vi "Teleop.vi"(10 "Match Info":T2={"Autonomous Elapsed Seconds"=0.0, "TeleOp Elapsed Seconds"=23.221, "Disabled Elapsed Seconds"=215.834, "Visited Autonomous"=FALSE, "Visited TeleOp"=TRUE, "Visited Disabled"=TRUE, "Autonomous Settings"={"Autonomous Style"=enum."Independent", "VI Refnum"=refnum}}, 11 "Call Context":T3=enum."Stop") -> ()   [LabVIEW 2016]
doc: "This VI is called for each TeleOp packet received from the DS where the robot is not disabled. It is often used to read from the joysticks and update I/O or to update setpoints for timed control loops. It should complete and return within 20 milliseconds or it may miss DS packets."
uses:
  <vilib>/Rock Robotics/WPI/DriverStation/WPI_DriverStationDerivedRobotMode.ctl
  <vilib>/Rock Robotics/WPI/DriverStation/WPI_DriverStationMatch Info.ctl
  <userlib>/836-libraries/Drive/Drive_Code/Drive_Code_Support/Drive_Code_PID_Bundle.ctl
  FMS Commands.ctl
  Drive Commands.ctl
  Gear Command.ctl
  <userlib>/836-libraries/Drive/Drive_Code/Drive_Code_Support/Sensor_Cluster.ctl
  <userlib>/836-libraries/Drive/Drive_Code/Drive_Code_Support/Camera_Cluster.ctl
  <userlib>/836-libraries/Drive/Drive_Code/Drive_Code_Support/Drive_Code_Notifier.ctl
  <userlib>/836-libraries/Drive/Drive_Code/Drive_Code_Support/Drive_Code_Command.ctl
  <userlib>/836-libraries/Drive/Drive_Code/Logging_Data.ctl
  <vilib>/Rock Robotics/WPI/Utilities/WPI_GetSetVariantRefNum.vi
panel:
  in  "Tab Control":enum32{"Drive", "Page 2"}(tab)
  in  "High Gear PID":T1={"Yaw, Driving Straight"={"proportional gain (Kc)"=1.0, "integral time (Ti, min)"=0.01, "derivative time (Td, min)"=0.0}, "Yaw, Holding Still"={"proportional gain (Kc)"=1.0, "integral time (Ti, min)"=0.01, "derivative time (Td, min)"=0.0}, "Distance, Driving Straight"={"proportional gain (Kc)"=1.0, "integral time (Ti, min)"=0.01, "derivative time (Td, min)"=0.0}, "Distance, Holding Still"={"proportional gain (Kc)"=1.0, "integral time (Ti, min)"=0.01, "derivative time (Td, min)"=0.0}}
  in  "Low Gear PID":T1={"Yaw, Driving Straight"={"proportional gain (Kc)"=1.0, "integral time (Ti, min)"=0.01, "derivative time (Td, min)"=0.0}, "Yaw, Holding Still"={"proportional gain (Kc)"=1.0, "integral time (Ti, min)"=0.01, "derivative time (Td, min)"=0.0}, "Distance, Driving Straight"={"proportional gain (Kc)"=1.0, "integral time (Ti, min)"=0.01, "derivative time (Td, min)"=0.0}, "Distance, Holding Still"={"proportional gain (Kc)"=1.0, "integral time (Ti, min)"=0.01, "derivative time (Td, min)"=0.0}}
  in  "PID Update":bool
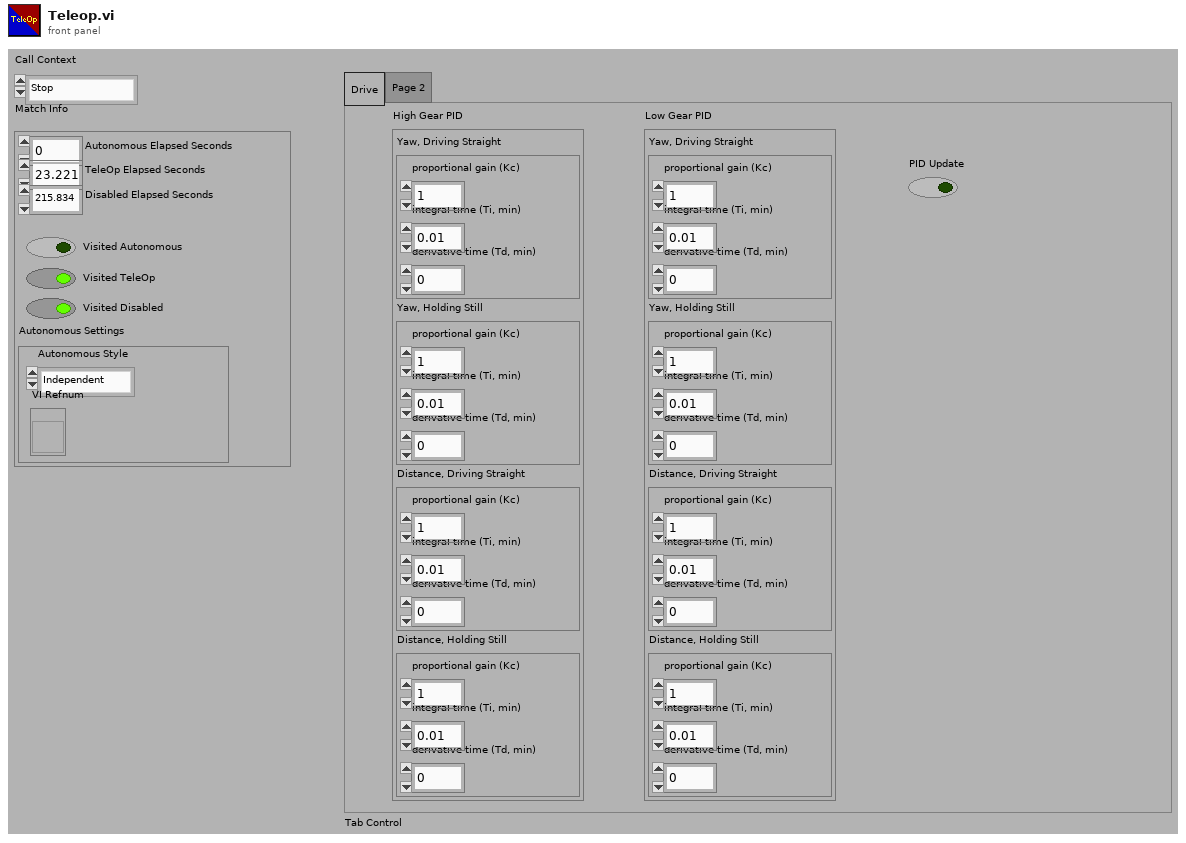
[diagram p1: front panel]
types:
  T1 = typedef "Drive_Code_PID_Bundle.ctl" = cluster{"Yaw, Driving Straight":cluster{"proportional gain (Kc)":dbl, "integral time (Ti, min)":dbl, "derivative time (Td, min)":dbl}, "Yaw, Holding Still":cluster{"proportional gain (Kc)":dbl, "integral time (Ti, min)":dbl, "derivative time (Td, min)":dbl}, "Distance, Driving Straight":cluster{"proportional gain (Kc)":dbl, "integral time (Ti, min)":dbl, "derivative time (Td, min)":dbl}, "Distance, Holding Still":cluster{"proportional gain (Kc)":dbl, "integral time (Ti, min)":dbl, "derivative time (Td, min)":dbl}}
  T2 = typedef "WPI_DriverStationMatch Info.ctl" = cluster{"Autonomous Elapsed Seconds":dbl, "TeleOp Elapsed Seconds":dbl, "Disabled Elapsed Seconds":dbl, "Visited Autonomous":bool, "Visited TeleOp":bool, "Visited Disabled":bool, "Autonomous Settings":cluster{"Autonomous Style":enum16{"Iterative", "Independent"}, "VI Refnum":refnum<vi>}}
  T3 = typedef "WPI_DriverStationDerivedRobotMode.ctl" = enum16{"Init", "Execute", "Stop"}
  T4 = typedef "WPI_JoystickDevRef.ctl" = cluster{"Device":T5}
  T5 = typedef "WPI_JoystickDeviceEnum.ctl" = enum16{"USB 0", "USB 1", "USB 2", "USB 3", "USB 4", "USB 5"}
  T6 = enum8{"setop", "setcolor", "default", "pilot", "ball", "gear", "both", "gearDeliver", "timeWarn", "targeting", "rave", "debug", "Set Power"}
  T7 = typedef "Sensor_Cluster.ctl" = cluster{"Gyro Data":cluster{"Gyro RT FIFO":refnum<k33>, "Gyro Current":dbl, "Gyro Hold":dbl}, "Encoder Data":cluster{"Encoder RT FIFO":refnum<k33>, "Encoder Current":dbl, "Encoder Hold":dbl}, "Camera Data":cluster{"Camera RT FIFO":refnum<k33>, "Camera Current":T8}}
  T8 = typedef "Camera_Cluster.ctl" = cluster{" Angle":dbl, "Valid":bool}
  T9 = cluster{"Cluster":T7, "Drive Command rt fifo":refnum<k33>, "Logging Data":refnum<k33>, "PID Update":refnum<notifier>}
  T10 = typedef "FMS Commands.ctl" = enum16{"Shoot", "Un-Jam", "Stop"}
  T11 = typedef "Gear Command.ctl" = enum16{"Home", "Floor Intake", "Catch", "Score"}
  T12 = typedef "Drive Commands.ctl" = enum16{"Manual", "Get Gear", "Score Gear", "Align Rope", "Turn To Angle", "Start Gear Score", "Place Gear", "Tank Drive", "Drive Distance"}
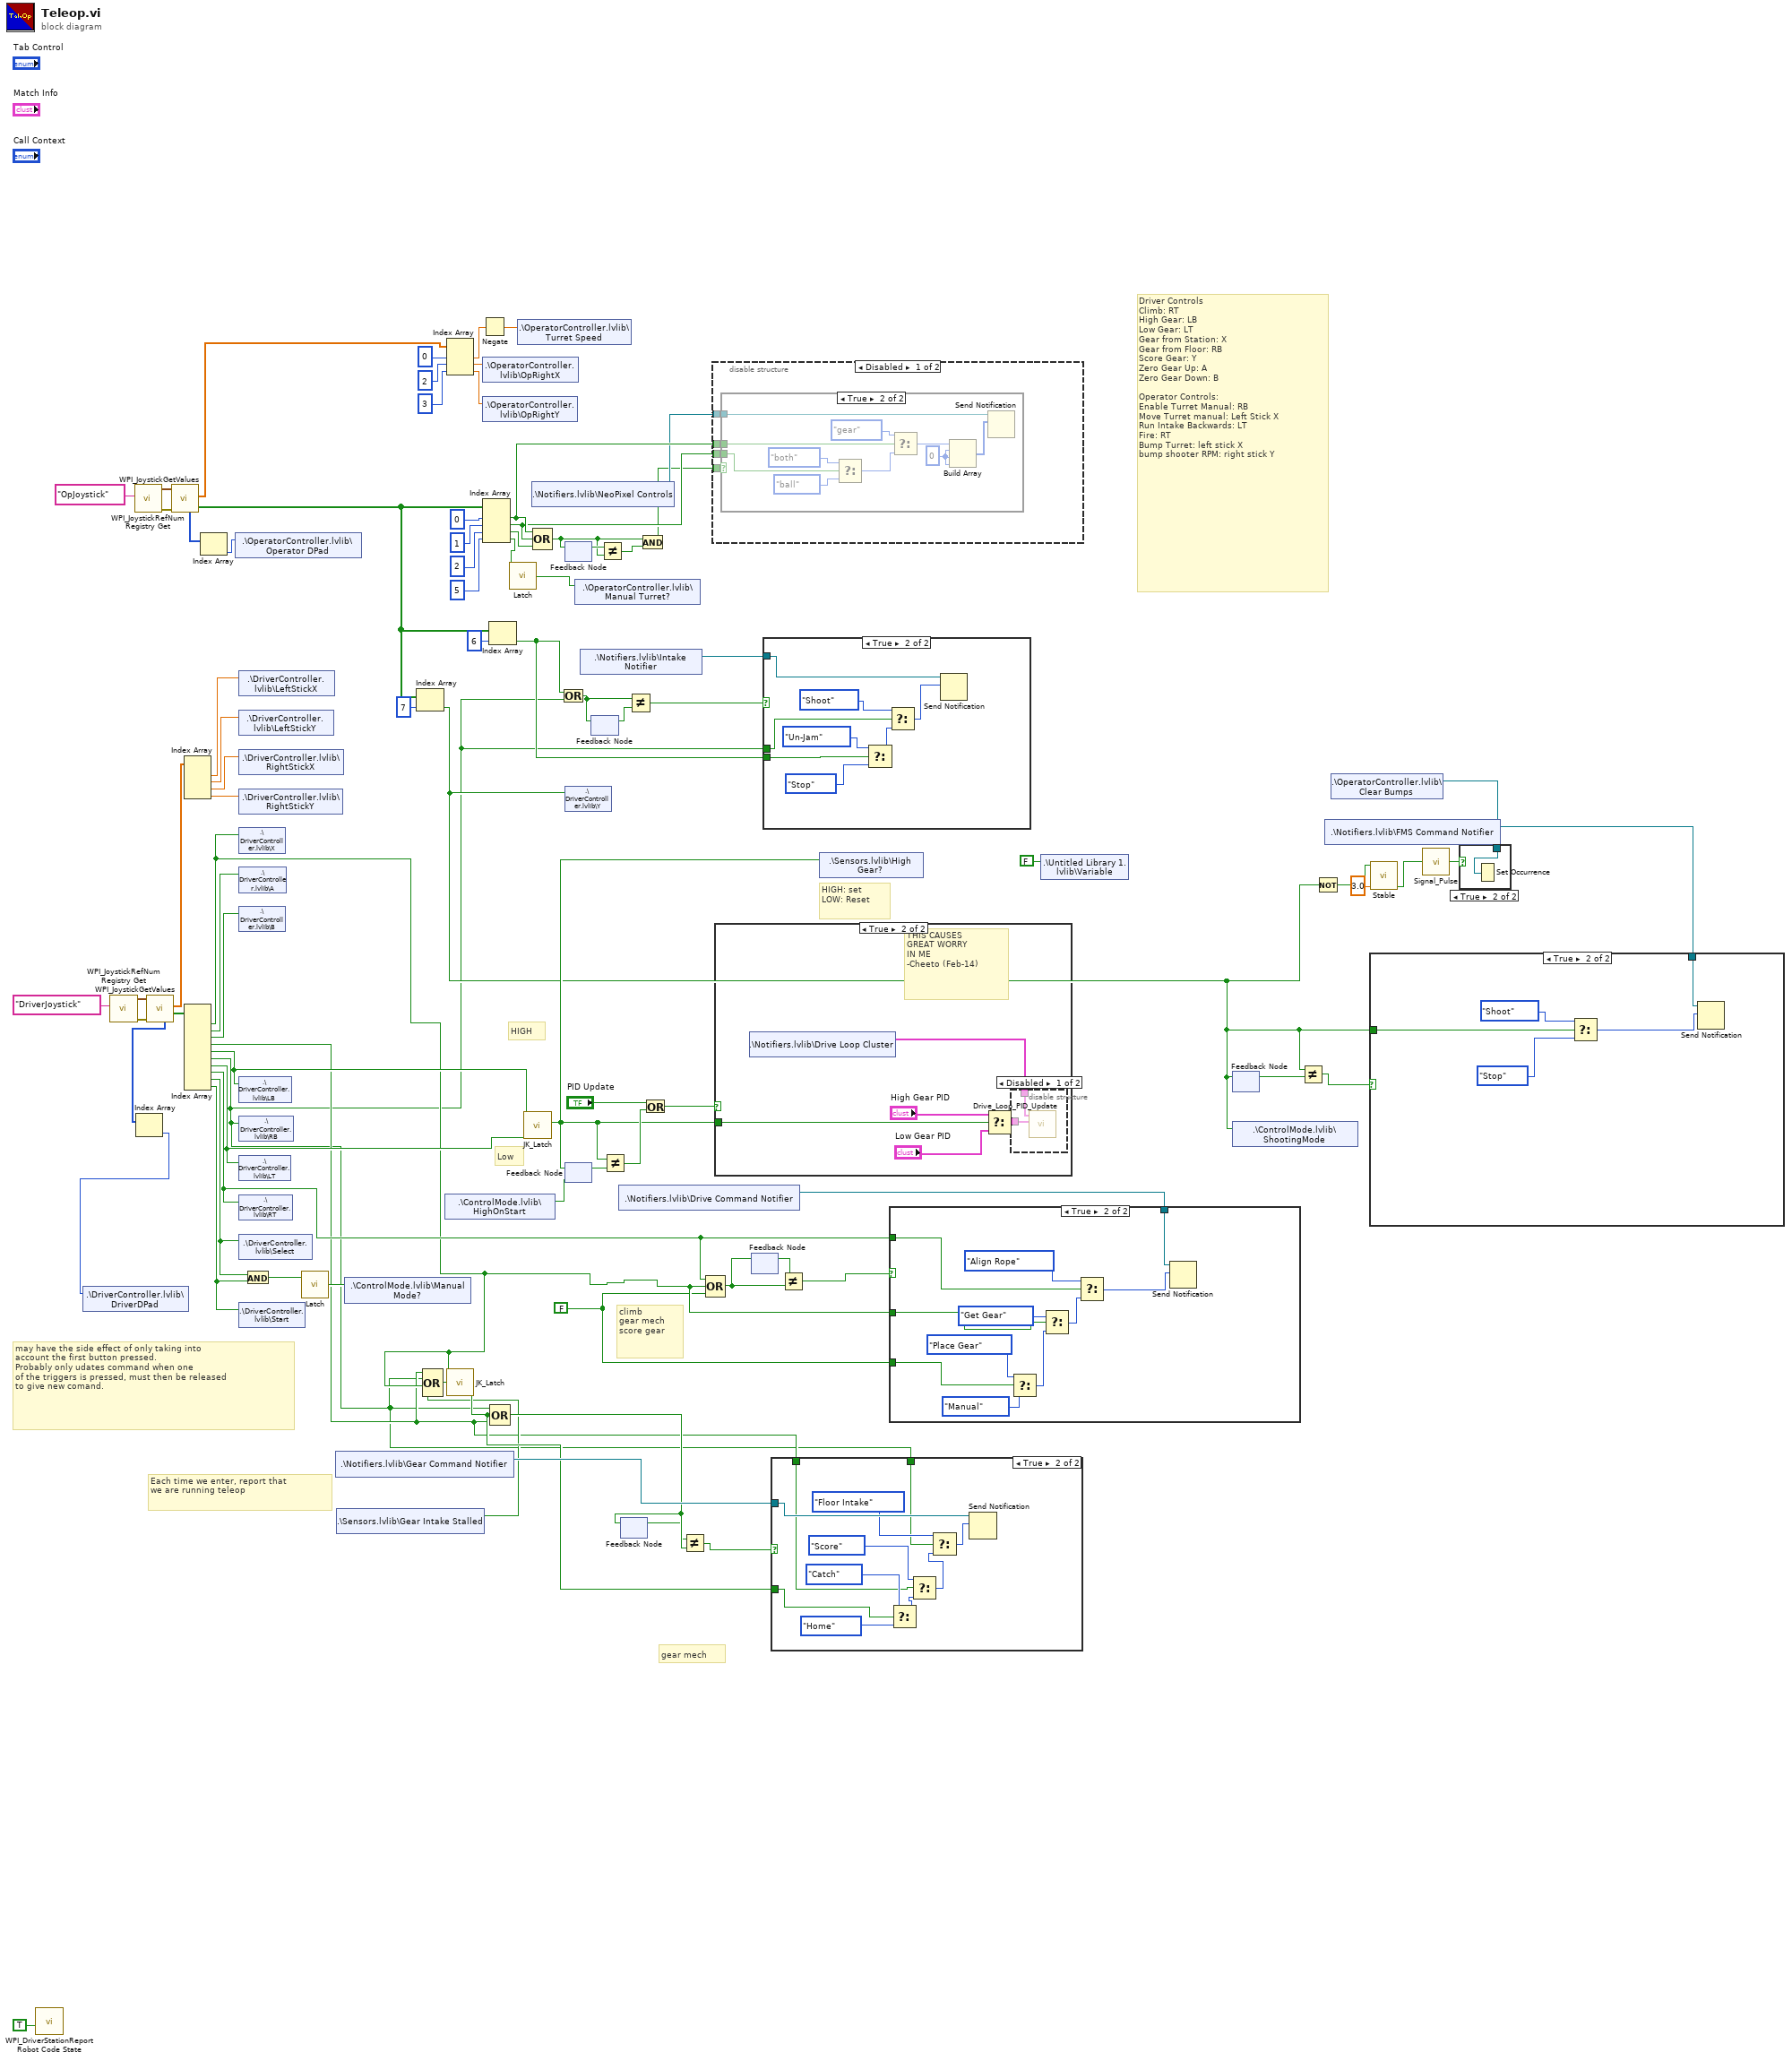
[diagram p0: block diagram]
diagram:
  w1 = FALSE ("value")
  # "climb\ngear mech\nscore gear"
  # "gear mech"
  # "HIGH: set\nLOW: Reset"
  # "Low"
  # "HIGH"
  # "Driver Controls\nClimb: RT\nHigh Gear: LB\nLow Gear: LT\nGear from Station: X\nGear from Floor: RB\nScore Gear: Y\nZero Gear Up: A\nZero Gear Down: B\n\nOperator Controls:\nEnable Turret Manual: RB\nMove Turret manual: Left Stick X\nRun Intake Backwards: LT\nFire: RT\nBump Turret: left stick X\nbump shooter RPM: right stick Y"
  # "may have the side effect of only taking into\naccount the first button pressed.\nProbably only udates command when one\nof the triggers is pressed, must then be released\nto give new comand."
  # "Each time we enter, report that\nwe are running teleop"
  n1 = call <vilib>:"WPI_DriverStationReport Robot Code State.vi"("TeleOp"=TRUE ("Autonomous")) -> ()  [unwired: 10 in, 1 out]
  n2 = call <vilib>:"WPI_JoystickRefNum Registry Get.vi"("refnum name"="DriverJoystick") -> ("error out"=w54:errorcluster, "JoystickDevRef"=w55:T4)  [unwired: 9 in]
  n3 = call <vilib>:"WPI_JoystickRefNum Registry Get.vi"("refnum name"="OpJoystick") -> ("error out"=w68:errorcluster, "JoystickDevRef"=w66:T4)  [unwired: 9 in]
  n4 = call <vilib>:"WPI_JoystickGetValues.vi"("error in (no error)"=w54, "JoystickDevRef"=w55) -> ("Buttons"=w84:bool[], "Axes"=w85:dbl[], "POVs"=w37:i16[])  [unwired: 5 in, 2 out]
  n5 = Index Array(array=w37) -> (element=w36:i16)  [unwired: 1 in]
  n6 = shared-variable ".\\DriverController.lvlib\\DriverDPad"(w36) -> ()  [unwired: 1 in, 1 out]
  n7 = call <vilib>:"WPI_JoystickGetValues.vi"("error in (no error)"=w68, "JoystickDevRef"=w66) -> ("Buttons"=w33:bool[], "Axes"=w65:dbl[], "POVs"=w35:i16[])  [unwired: 5 in, 2 out]
  n8 = Index Array(array=w85) -> (element #1=w83:dbl, element #2=w74:dbl, element #3=w73:dbl, element #4=w82:dbl)  [unwired: 4 in]
  n9 = Index Array(array=w84) -> (element #1=w4:bool, element #2=w14:bool, element #3=w69:bool, element #4=w3:bool, element #5=w48:bool, element #6=w2:bool, element #7=w47:bool, element #8=w15:bool, element #9=w78:bool, element #10=w77:bool)  [unwired: 10 in]
  n10 = Index Array(array=w35) -> (element=w34:i16)  [unwired: 1 in]
  n11 = shared-variable ".\\OperatorController.lvlib\\Operator DPad"(w34) -> ()  [unwired: 1 in, 1 out]
  n12 = shared-variable ".\\DriverController.lvlib\\LeftStickX"(w83) -> ()  [unwired: 1 in, 1 out]
  n13 = shared-variable ".\\DriverController.lvlib\\LeftStickY"(w74) -> ()  [unwired: 1 in, 1 out]
  n14 = shared-variable ".\\DriverController.lvlib\\RightStickX"(w73) -> ()  [unwired: 1 in, 1 out]
  n15 = shared-variable ".\\DriverController.lvlib\\RightStickY"(w82) -> ()  [unwired: 1 in, 1 out]
  n16 = shared-variable ".\\DriverController.lvlib\\X"(w4) -> ()  [unwired: 1 in, 1 out]
  n17 = shared-variable ".\\DriverController.lvlib\\A"(w14) -> ()  [unwired: 1 in, 1 out]
  n18 = shared-variable ".\\DriverController.lvlib\\B"(w69) -> ()  [unwired: 1 in, 1 out]
  n19 = shared-variable ".\\DriverController.lvlib\\LB"(w48) -> ()  [unwired: 1 in, 1 out]
  n20 = shared-variable ".\\DriverController.lvlib\\RB"(w2) -> ()  [unwired: 1 in, 1 out]
  n21 = shared-variable ".\\DriverController.lvlib\\LT"(w47) -> ()  [unwired: 1 in, 1 out]
  n22 = shared-variable ".\\DriverController.lvlib\\RT"(w15) -> ()  [unwired: 1 in, 1 out]
  n23 = shared-variable ".\\DriverController.lvlib\\Select"(w78) -> ()  [unwired: 1 in, 1 out]
  n24 = shared-variable ".\\DriverController.lvlib\\Start"(w77) -> ()  [unwired: 1 in, 1 out]
  n25 = And(x=w78, y=w77) -> (x .and. y?=w76:bool)
  n26 = call <userlib>:"Latch.vi"("In"=w76) -> ("Out"=w70:bool)  [unwired: 1 in]
  n27 = shared-variable ".\\Notifiers.lvlib\\Gear Command Notifier"() -> (w11:refnum<notifier>)  [unwired: 1 in, 1 out]
  n28 = shared-variable ".\\Sensors.lvlib\\Gear Intake Stalled"() -> (w5:bool)  [unwired: 1 in, 1 out]
  n29 = shared-variable ".\\ControlMode.lvlib\\Manual Mode?"(w70) -> ()  [unwired: 1 in, 1 out]
  n30 = Index Array(array=w33, index=7) -> (element=w12:bool)
  n31 = Compound Arithmetic op=OR(w3, w2, w4, w5) -> (w6:bool)
  n32 = shared-variable ".\\ControlMode.lvlib\\HighOnStart"() -> (w75:bool)  [unwired: 1 in, 1 out]
  n33 = Index Array(array=w65, index #1=0 ("index"), index #2=2 ("index"), index #3=3 ("index")) -> (element #1=w50:dbl, element #2=w26:dbl, element #3=w25:dbl)
  n34 = call <userlib>:"JK_Latch.vi"("Reset"=w6, "Set"=w4) -> ("Q"=w7:bool)  [unwired: 5 in]
  n35 = Negate(x=w50) -> (-x=w49:dbl)
  n36 = shared-variable ".\\OperatorController.lvlib\\OpRightX"(w26) -> ()  [unwired: 1 in, 1 out]
  n37 = shared-variable ".\\OperatorController.lvlib\\OpRightY"(w25) -> ()  [unwired: 1 in, 1 out]
  n38 = Index Array(array=w33, index #1=0 ("index"), index #2=1 ("index"), index #3=2 ("index"), index #4=5 ("index")) -> (element #1=w58:bool, element #2=w57:bool, element #3=w60:bool, element #4=w30:bool)
  n39 = Index Array(array=w33, index=6) -> (element=w41:bool)
  n40 = Compound Arithmetic op=OR(w2, w7, w3) -> (w10:bool)
  n41 = call <userlib>:"Latch.vi"("In"=w30) -> ("Out"=w31:bool)  [unwired: 1 in]
  n42 = shared-variable ".\\OperatorController.lvlib\\Turret Speed"(w49) -> ()  [unwired: 1 in, 1 out]
  n43 = call <userlib>:"JK_Latch.vi"("Reset"=w47, "Set"=w48) -> ("Q"=w79:bool)  [unwired: 5 in]
  n44 = shared-variable ".\\Notifiers.lvlib\\NeoPixel Controls"() -> (w56:refnum<notifier>)  [unwired: 1 in, 1 out]
  n45 = Compound Arithmetic op=OR(w58, w57, w60) -> (w51:bool)
  n46 = Or(x=w41, y=w2) -> (x .or. y?=w45:bool)
  n47 = feedback-in #1(w51) -> ()
  n48 = feedback #1() -> (w59:bool)  [unwired: 1 in]
  n49 = shared-variable ".\\DriverController.lvlib\\Y"(w12) -> ()  [unwired: 1 in, 1 out]
  n50 = feedback-in #2(w79) -> ()
  n51 = feedback #2(w75) -> (w81:bool)
  n52 = shared-variable ".\\OperatorController.lvlib\\Manual Turret?"(w31) -> ()  [unwired: 1 in, 1 out]
  n53 = shared-variable ".\\Notifiers.lvlib\\Intake Notifier"() -> (w42:refnum<notifier>)  [unwired: 1 in, 1 out]
  n54 = feedback-in #3(w45) -> ()
  n55 = feedback #3() -> (w44:bool)  [unwired: 1 in]
  n56 = Not Equal?(x=w59, y=w51) -> (x != y?=w53:bool)
  n57 = Not Equal?(x=w79, y=w81) -> (x != y?=w80:bool)
  n58 = shared-variable ".\\Notifiers.lvlib\\Drive Command Notifier"() -> (w13:refnum<notifier>)  [unwired: 1 in, 1 out]
  n59 = feedback-in #4(w10) -> ()
  n60 = feedback #4() -> (w9:bool)  [unwired: 1 in]
  n61 = Not Equal?(x=w45, y=w44) -> (x != y?=w43:bool)
  n62 = And(x=w51, y=w53) -> (x .and. y?=w52:bool)
  n63 = Or(x="PID Update", y=w80) -> (x .or. y?=w72:bool)
  n64 = Not Equal?(x=w9, y=w10) -> (x != y?=w8:bool)
  n65 = Compound Arithmetic op=OR(w15, w4, w1) -> (w17:bool)
  n66 = disable-structure shown="Disabled" {
    disable-tunnel: w58 -> [w91 _]
    disable-tunnel: w57 -> [w90 _]
    disable-tunnel: w56 -> [w89 _]
    disable-tunnel: w52 -> [w88 _]
    frame Disabled {
      n67 = case shown="True" w88 {
        tunnel: w91 -> [_ w98]
        tunnel: w90 -> [_ w101]
        tunnel: w89 -> [_ w100]
        frame False {
        }
        frame True {
          w92 = 0
          n68 = Select(t=T6."both" ("Enum"), s=w101, f=T6."ball" ("Enum")) -> (s? t:f=w99:T6)
          n69 = Select(t=T6."gear" ("Enum"), s=w98, f=w99) -> (s? t:f=w94:T6)
          n70 = Build Array(w94, w92, w92, w92) -> (w93:i32[])
          n71 = Send Notification(notification=w93, notifier=w100) -> ()  [unwired: 1 in, 2 out]
        }
      }
    }
    frame Enabled {
    }
  }
  n72 = case shown="True" w72 {
    tunnel: w79 -> [_ w106]
    frame False {
    }
    frame True {
      # "THIS CAUSES\nGREAT WORRY\nIN ME\n-Cheeto (Feb-14)"
      n73 = shared-variable ".\\Notifiers.lvlib\\Drive Loop Cluster"() -> (w102:T9)  [unwired: 1 in, 1 out]
      n74 = Select(t="High Gear PID", s=w106, f="Low Gear PID") -> (s? t:f=w103:T1)
      n75 = disable-structure shown="Disabled" {
        disable-tunnel: w103 -> [w108 _]
        disable-tunnel: w102 -> [w107 _]
        frame Disabled {
          n76 = call <userlib>:"Drive_Loop_PID_Update.vi"("PID Gains"=w108, "Control Cluster"=w107) -> ()  [unwired: 10 in]
        }
        frame Enabled {
        }
      }
    }
  }
  n77 = feedback-in #5(w17) -> ()
  n78 = feedback #5() -> (w18:bool)  [unwired: 1 in]
  n79 = case shown="True" w43 {
    tunnel: w42 -> [_ w116]
    tunnel: w2 -> [_ w114]
    tunnel: w41 -> [_ w113]
    frame False {
    }
    frame True {
      n80 = Select(t=FMS_Commands."Un-Jam", s=w113, f=FMS_Commands."Stop") -> (s? t:f=w111:T10)
      n81 = Select(t=FMS_Commands."Shoot", s=w114, f=w111) -> (s? t:f=w110:T10)
      n82 = Send Notification(notification=w110, notifier=w116) -> ()  [unwired: 1 in, 2 out]
    }
  }
  n83 = case shown="True" w8 {
    tunnel: w11 -> [_ w127]
    tunnel: w2 -> [_ w119]
    tunnel: w7 -> [_ w117]
    tunnel: w3 -> [_ w118]
    frame False {
    }
    frame True {
      n84 = Select(t=Gear_Command."Catch", s=w117, f=Gear_Command."Home") -> (s? t:f=w123:T11)
      n85 = Select(t=Gear_Command."Score", s=w118, f=w123) -> (s? t:f=w124:T11)
      n86 = Select(t=Gear_Command."Floor Intake", s=w119, f=w124) -> (s? t:f=w126:T11)
      n87 = Send Notification(notification=w126, notifier=w127) -> ()  [unwired: 1 in, 2 out]
    }
  }
  n88 = Not Equal?(x=w18, y=w17) -> (x != y?=w16:bool)
  n89 = shared-variable ".\\Sensors.lvlib\\High Gear?"(w79) -> ()  [unwired: 1 in, 1 out]
  n90 = case shown="True" w16 {
    tunnel: w15 -> [_ w137]
    tunnel: w4 -> [_ w135]
    tunnel: w1 -> [_ w133]
    tunnel: w13 -> [_ w138]
    frame False {
    }
    frame True {
      n91 = Select(t=Drive_Commands."Place Gear" ("notification"), s=w133, f=Drive_Commands."Manual" ("notification")) -> (s? t:f=w130:T12)
      n92 = Select(t=Drive_Commands."Get Gear" ("notification"), s=w135, f=w130) -> (s? t:f=w129:T12)
      n93 = Select(t=Drive_Commands."Align Rope" ("notification"), s=w137, f=w129) -> (s? t:f=w128:T12)
      n94 = Send Notification(notification=w128, notifier=w138) -> ()  [unwired: 1 in, 2 out]
    }
  }
  n95 = shared-variable ".\\Untitled Library 1.lvlib\\Variable"(FALSE ("Variable")) -> ()  [unwired: 1 in, 1 out]
  n96 = feedback-in #6(w12) -> ()
  n97 = feedback #6() -> (w38:bool)  [unwired: 1 in]
  n98 = shared-variable ".\\ControlMode.lvlib\\ShootingMode"(w12) -> ()  [unwired: 1 in, 1 out]
  n99 = Not Equal?(x=w12, y=w38) -> (x != y?=w39:bool)
  n100 = Not(x=w12) -> (.not. x?=w24:bool)
  n101 = shared-variable ".\\Notifiers.lvlib\\FMS Command Notifier"() -> (w40:refnum<notifier>)  [unwired: 1 in, 1 out]
  n102 = shared-variable ".\\OperatorController.lvlib\\Clear Bumps"() -> (w21:refnum<k4>)  [unwired: 1 in, 1 out]
  n103 = case shown="True" w39 {
    tunnel: w40 -> [_ w143]
    tunnel: w12 -> [_ w139]
    frame False {
    }
    frame True {
      n104 = Select(t=FMS_Commands."Shoot" ("notification"), s=w139, f=FMS_Commands."Stop" ("notification")) -> (s? t:f=w140:T10)
      n105 = Send Notification(notification=w140, notifier=w143) -> ()  [unwired: 1 in, 2 out]
    }
  }
  n106 = call <userlib>:"Stable.vi"("Eval Period (sec)"=3.0, "Signal Input"=w24) -> ("Stable"=w22:bool)  [unwired: 9 in]
  n107 = call <userlib>:"Signal_Pulse.vi"("Input"=w22) -> ("Output"=w20:bool)
  n108 = case shown="True" w20 {
    tunnel: w21 -> [_ w144]
    frame False {
    }
    frame True {
      n109 = Set Occurrence(w144) -> ()
    }
  }
